vi "白子权值.vi"(0 "当前棋盘状态":i32[][](array[numeric]), 7 "行":dbl, 9 "列":u8) -> (4 "白子总权值":i32)   [LabVIEW 2018]
panel:
  out "活1?右上":bool
  out "活1?左下":bool
  out "活1?左上":bool
  out "活1?右下":bool
  out "活1?正上":bool
  out "活1?正下":bool
  out "活1?正左":bool
  out "活1?正右":bool
  out "3个白子？右上":bool
  out "2个白子？右上":bool
  out "1个白子？右上":bool
  out "3个白子？左下":bool
  out "2个白子？左下":bool
  out "1个白子？ 左下":bool
  out "3个白子？左上":bool
  out "2个白子？左上":bool
  out "1个白子？左上":bool
  out "3个白子？右下":bool
  out "2个白子？右下":bool
  out "1个白子？右下":bool
  out "3个白子？ 正上":bool
  out "2个白子？ 正上":bool
  out "1个白子？ 正上":bool
  out "3个白子？ 正下":bool
  out "2个白子？正下":bool
  out "1个白子？ 正下":bool
  out "3个白子？正左":bool
  out "2个白子？正左":bool
  out "1个白子？正左":bool
  out "3个白子？正右":bool
  out "2个白子？正右":bool
  out "1个白子？正右":bool
  out "右上方向权值":i32
  out "左下方向权值":i32
  out "左上方向权值":i32
  out "右下方向权值":i32
  out "正上方权值":i32
  out "正下方权值":i32
  out "正左方向权值":i32
  out "正右方向权值":i32
  # "0"
  # "1"
  # "2"
  # "3"
  # "4"
  # "5"
  # "6"
  # "7"
  # "8"
  # "9"
  # "10"
  # "11"
  # "12"
  # "13"
  # "14"
  # "0"
  # "1"
  # "2"
  # "3"
  # "4"
  # "5"
  # "6"
  # "7"
  # "8"
  # "9"
  # "10"
  # "11"
  # "12"
  # "13"
  # "14"
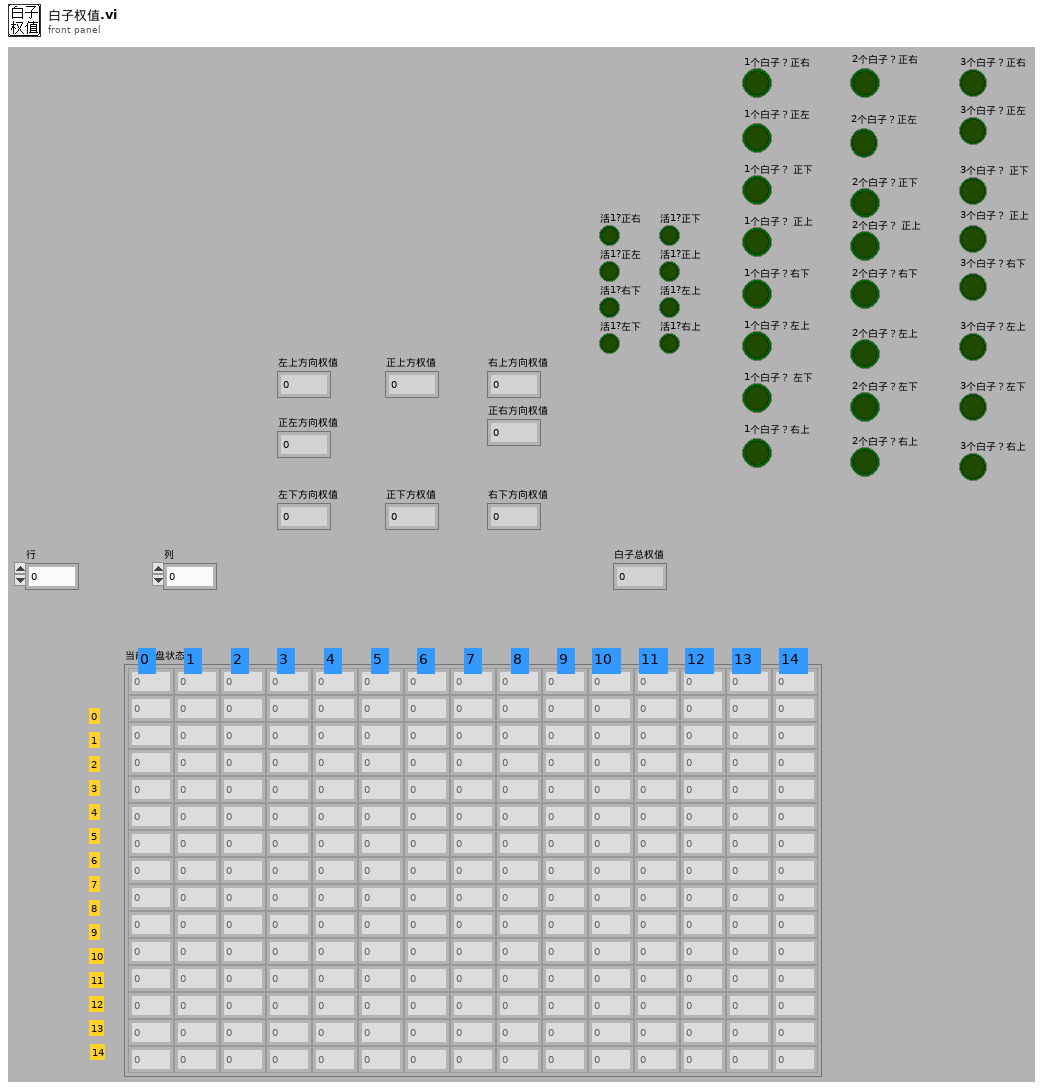
[diagram p1: front panel]
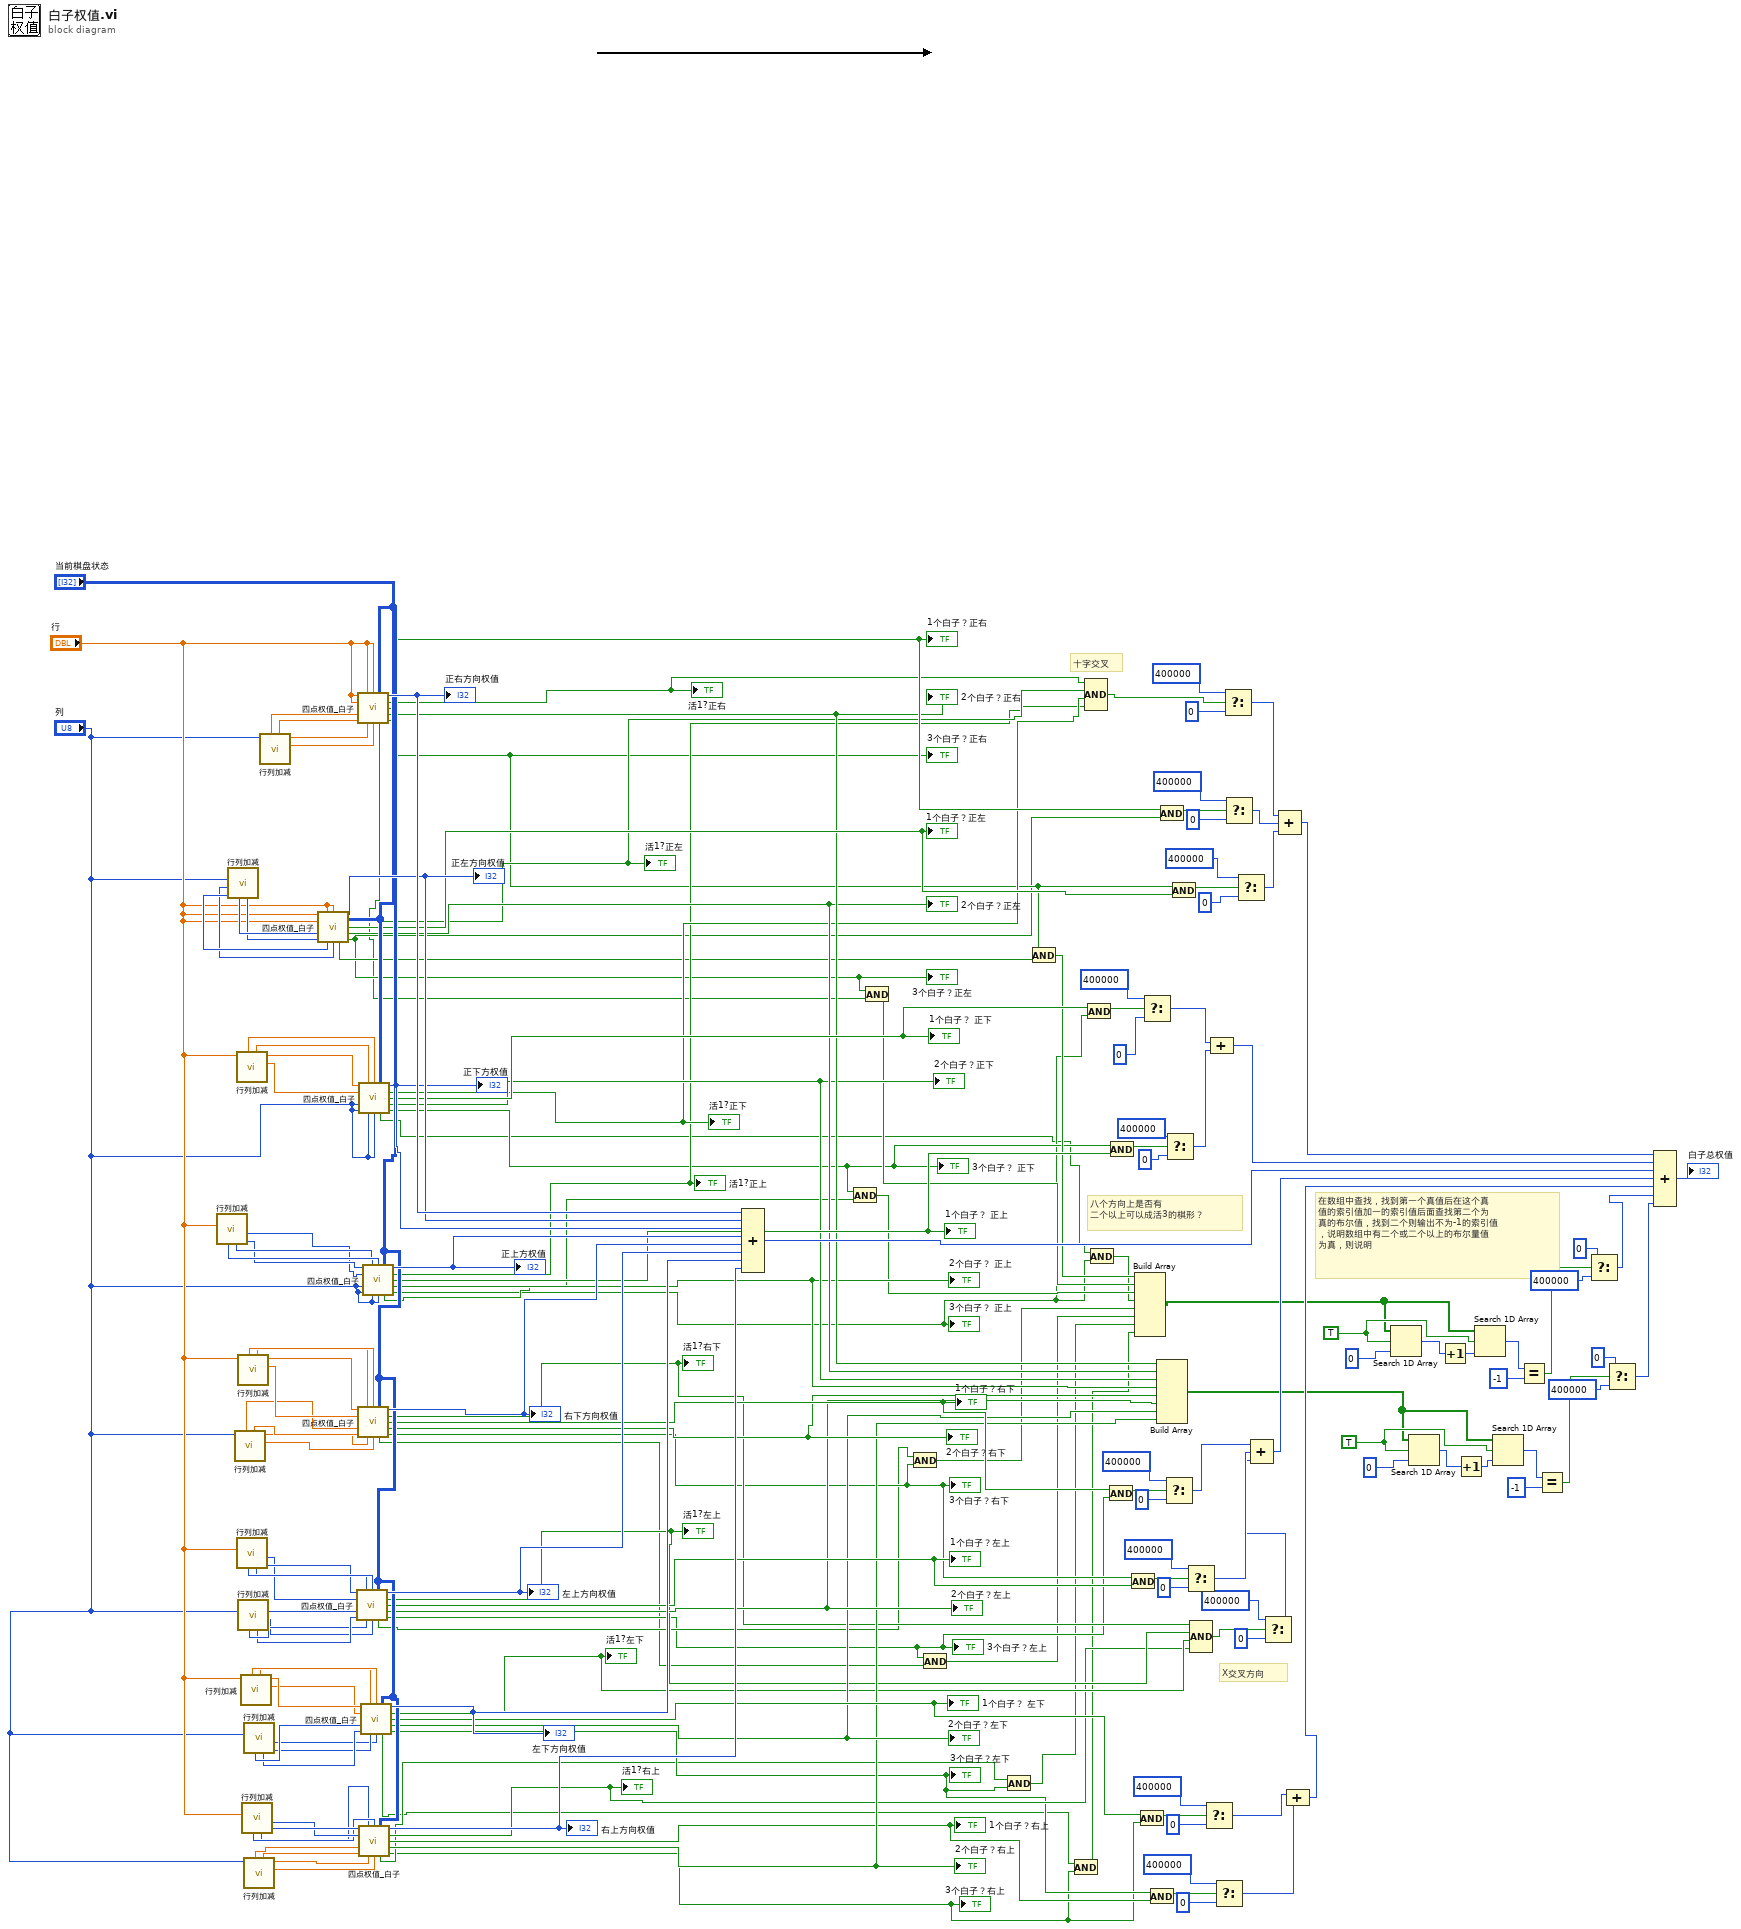
[diagram p0: block diagram]
diagram:
  w49 = TRUE ("element")
  w72 = TRUE ("element")
  # "在数组中查找，找到第一个真值后在这个真\n值的索引值加一的索引值后面查找第二个为\n真的布尔值，找到二个则输出不为-1的索引值\n，说明数组中有二个或二个以上的布尔量值\n为真，则说明"
  # "八个方向上是否有\n二个以上可以成活3的棋形？"
  # "X交叉方向"
  # "十字交叉"
  n1 = call "行列加减.vi"("减"="行") -> ("x-3"=w157:i32, "x-4"=w156:i32, "x-2"=w158:i32, "x-1"=w159:i32)  [unwired: 3 in, 4 out]
  n2 = call "行列加减.vi"("减"="列") -> ("x-3"=w165:i32, "x-4"=w164:i32, "x-2"=w166:i32, "x-1"=w167:i32)  [unwired: 3 in, 4 out]
  n3 = call "行列加减.vi"("加"="列") -> ("x+4"=w148:dbl, "x+3"=w149:dbl, "x+2"=w150:dbl, "x+1"=w151:dbl)  [unwired: 3 in, 4 out]
  n4 = call "行列加减.vi"("加"="行") -> ("x+4"=w160:dbl, "x+3"=w161:dbl, "x+2"=w162:dbl, "x+1"=w163:dbl)  [unwired: 3 in, 4 out]
  n5 = call "行列加减.vi"("减"="行") -> ("x-3"=w144:i32, "x-4"=w143:i32, "x-2"=w145:i32, "x-1"=w146:i32)  [unwired: 3 in, 4 out]
  n6 = call "行列加减.vi"("加"="行") -> ("x+4"=w152:dbl, "x+3"=w153:dbl, "x+2"=w154:dbl, "x+1"=w155:dbl)  [unwired: 3 in, 4 out]
  n7 = call "行列加减.vi"("减"="列") -> ("x-3"=w140:i32, "x-4"=w139:i32, "x-2"=w141:i32, "x-1"=w142:i32)  [unwired: 3 in, 4 out]
  n8 = call "行列加减.vi"("加"="行") -> ("x+4"=w134:dbl, "x+3"=w135:dbl, "x+2"=w136:dbl, "x+1"=w137:dbl)  [unwired: 3 in, 4 out]
  n9 = call "行列加减.vi"("减"="行") -> ("x-3"=w125:i32, "x-4"=w124:i32, "x-2"=w117:i32, "x-1"=w118:i32)  [unwired: 3 in, 4 out]
  n10 = call "行列加减.vi"("减"="列") -> ("x-3"=w131:i32, "x-4"=w130:i32, "x-2"=w132:i32, "x-1"=w133:i32)  [unwired: 3 in, 4 out]
  n11 = call "行列加减.vi"("加"="列") -> ("x+4"=w120:dbl, "x+3"=w121:dbl, "x+2"=w122:dbl, "x+1"=w123:dbl)  [unwired: 3 in, 4 out]
  n12 = call "行列加减.vi"("加"="列") -> ("x+4"=w168:dbl, "x+3"=w169:dbl, "x+2"=w170:dbl, "x+1"=w171:dbl)  [unwired: 3 in, 4 out]
  n13 = call "四点权值_白子.vi"("3位置行"="行", "2位置行"="行", "1位置行"="行", "当前棋盘状态"="当前棋盘状态", "4位置行"="行", "1位置列"=w167, "2位置列"=w166, "3位置列"=w165, "4位置列"=w164) -> ("白子四位置权值"=w174:i32, "有2个白子?或白子加无子?"=w41:bool, "第1个是白子？"=w108:bool, "3个白子?"=w61:bool, "第一个位置为空？"=w23:bool, "3个白子？或2个白子加无子"=w21:bool)  [unwired: 1 in]
  "正左方向权值" <- w174
  "1个白子？正左" <- w108
  "2个白子？正左" <- w61
  "3个白子？正左" <- w21
  "活1?正左" <- w41
  n14 = call "四点权值_白子.vi"("3位置行"=w144, "2位置行"=w145, "1位置行"=w146, "当前棋盘状态"="当前棋盘状态", "4位置行"=w143, "1位置列"=w142, "2位置列"=w141, "3位置列"=w140, "4位置列"=w139) -> ("白子四位置权值"=w138:i32, "有2个白子?或白子加无子?"=w33:bool, "第1个是白子？"=w86:bool, "3个白子?"=w57:bool, "第一个位置为空？"=w14:bool, "3个白子？或2个白子加无子"=w12:bool)  [unwired: 1 in]
  "左上方向权值" <- w138
  "1个白子？左上" <- w86
  "2个白子？左上" <- w57
  "3个白子？左上" <- w12
  "活1?左上" <- w33
  n15 = call "四点权值_白子.vi"("3位置行"="行", "2位置行"="行", "1位置行"="行", "当前棋盘状态"="当前棋盘状态", "4位置行"="行", "1位置列"=w171, "2位置列"=w170, "3位置列"=w169, "4位置列"=w168) -> ("白子四位置权值"=w175:i32, "有2个白子?或白子加无子?"=w26:bool, "第1个是白子？"=w112:bool, "3个白子?"=w62:bool, "第一个位置为空？"=w20:bool, "3个白子？或2个白子加无子"=w24:bool)  [unwired: 1 in]
  "正右方向权值" <- w175
  "1个白子？正右" <- w112
  "2个白子？正右" <- w62
  "3个白子？正右" <- w24
  "活1?正右" <- w26
  n16 = call "四点权值_白子.vi"("3位置行"=w153, "2位置行"=w154, "1位置行"=w155, "当前棋盘状态"="当前棋盘状态", "4位置行"=w152, "1位置列"=w151, "2位置列"=w150, "3位置列"=w149, "4位置列"=w148) -> ("白子四位置权值"=w147:i32, "有2个白子?或白子加无子?"=w34:bool, "第1个是白子？"=w91:bool, "3个白子?"=w58:bool, "第一个位置为空？"=w11:bool, "3个白子？或2个白子加无子"=w15:bool)  [unwired: 1 in]
  "右下方向权值" <- w147
  "1个白子？右下" <- w91
  "2个白子？右下" <- w58
  "3个白子？右下" <- w15
  "活1?右下" <- w34
  n17 = call "四点权值_白子.vi"("3位置行"=w161, "2位置行"=w162, "1位置行"=w163, "当前棋盘状态"="当前棋盘状态", "4位置行"=w160, "1位置列"="列", "2位置列"="列", "3位置列"="列", "4位置列"="列") -> ("白子四位置权值"=w173:i32, "有2个白子?或白子加无子?"=w40:bool, "第1个是白子？"=w102:bool, "3个白子?"=w60:bool, "第一个位置为空？"=w1:bool, "3个白子？或2个白子加无子"=w18:bool)  [unwired: 1 in]
  "正下方权值" <- w173
  "1个白子？ 正下" <- w102
  "2个白子？正下" <- w60
  "3个白子？ 正下" <- w18
  "活1?正下" <- w40
  n18 = call "四点权值_白子.vi"("3位置行"=w125, "2位置行"=w117, "1位置行"=w118, "当前棋盘状态"="当前棋盘状态", "4位置行"=w124, "1位置列"=w123, "2位置列"=w122, "3位置列"=w121, "4位置列"=w120) -> ("白子四位置权值"=w119:i32, "有2个白子?或白子加无子?"=w31:bool, "第1个是白子？"=w25:bool, "3个白子?"=w55:bool, "第一个位置为空？"=w7:bool, "3个白子？或2个白子加无子"=w6:bool)  [unwired: 1 in]
  "右上方向权值" <- w119
  "1个白子？右上" <- w25
  "2个白子？右上" <- w55
  "3个白子？右上" <- w6
  "活1?右上" <- w31
  n19 = call "四点权值_白子.vi"("3位置行"=w135, "2位置行"=w136, "1位置行"=w137, "当前棋盘状态"="当前棋盘状态", "4位置行"=w134, "1位置列"=w133, "2位置列"=w132, "3位置列"=w131, "4位置列"=w130) -> ("白子四位置权值"=w129:i32, "有2个白子?或白子加无子?"=w32:bool, "第1个是白子？"=w79:bool, "3个白子?"=w56:bool, "第一个位置为空？"=w5:bool, "3个白子？或2个白子加无子"=w8:bool)  [unwired: 1 in]
  "左下方向权值" <- w129
  "1个白子？ 左下" <- w79
  "2个白子？左下" <- w56
  "3个白子？左下" <- w8
  "活1?左下" <- w32
  n20 = call "四点权值_白子.vi"("3位置行"=w157, "2位置行"=w158, "1位置行"=w159, "当前棋盘状态"="当前棋盘状态", "4位置行"=w156, "1位置列"="列", "2位置列"="列", "3位置列"="列", "4位置列"="列") -> ("白子四位置权值"=w172:i32, "有2个白子?或白子加无子?"=w39:bool, "第1个是白子？"=w98:bool, "3个白子?"=w59:bool, "第一个位置为空？"=w17:bool, "3个白子？或2个白子加无子"=w2:bool)  [unwired: 1 in]
  "正上方权值" <- w172
  "1个白子？ 正上" <- w98
  "2个白子？ 正上" <- w59
  "3个白子？ 正上" <- w2
  "活1?正上" <- w39
  n21 = Compound Arithmetic op=ADD(w175, w174, w173, w172, w147, w138, w129, w119) -> (w95:i32)
  n22 = And(x=w18, y=w17) -> (x .and. y?=w16:bool)
  n23 = And(x=w21, y=w20) -> (x .and. y?=w19:bool)
  n24 = And(x=w14, y=w15) -> (x .and. y?=w13:bool)
  n25 = And(x=w12, y=w11) -> (x .and. y?=w10:bool)
  n26 = And(x=w7, y=w8) -> (x .and. y?=w9:bool)
  n27 = And(x=w24, y=w23) -> (x .and. y?=w22:bool)
  n28 = And(x=w5, y=w6) -> (x .and. y?=w4:bool)
  n29 = And(x=w102, y=w2) -> (x .and. y?=w105:bool)
  n30 = Compound Arithmetic op=AND(w26, w41, w40, w39) -> (w36:bool)
  n31 = And(x=w1, y=w2) -> (x .and. y?=w3:bool)
  n32 = And(x=w91, y=w12) -> (x .and. y?=w92:bool)
  n33 = And(x=w18, y=w98) -> (x .and. y?=w101:bool)
  n34 = And(x=w15, y=w86) -> (x .and. y?=w89:bool)
  n35 = Build Array(w22, w19, w16, w3, w13, w10, w9, w4) -> (w69:bool[])
  n36 = And(x=w79, y=w6) -> (x .and. y?=w83:bool)
  n37 = Select(t=400000, s=w105, f=0) -> (s? t:f=w63:i32)
  n38 = And(x=w8, y=w25) -> (x .and. y?=w75:bool)
  n39 = And(x=w112, y=w21) -> (x .and. y?=w114:bool)
  n40 = Build Array(w62, w61, w60, w59, w58, w57, w56, w55) -> (w47:bool[])
  n41 = Select(t=400000, s=w92, f=0) -> (s? t:f=w90:i32)
  n42 = Select(t=400000, s=w101, f=0) -> (s? t:f=w97:i32)
  n43 = And(x=w24, y=w108) -> (x .and. y?=w111:bool)
  n44 = Select(t=400000, s=w89, f=0) -> (s? t:f=w85:i32)
  n45 = Compound Arithmetic op=AND(w34, w33, w32, w31) -> (w29:bool)
  n46 = Select(t=400000, s=w83, f=0) -> (s? t:f=w78:i32)
  n47 = Compound Arithmetic op=ADD(w63, w97) -> (w96:i32)
  n48 = Select(t=400000, s=w75, f=0) -> (s? t:f=w74:i32)
  n49 = Select(t=400000, s=w36, f=0) -> (s? t:f=w35:i32)
  n50 = Select(t=400000, s=w114, f=0) -> (s? t:f=w113:i32)
  n51 = Select(t=400000, s=w111, f=0) -> (s? t:f=w107:i32)
  n52 = Select(t=400000, s=w29, f=0) -> (s? t:f=w27:i32)
  n53 = Compound Arithmetic op=ADD(w90, w85, w27) -> (w84:i32)
  n54 = Compound Arithmetic op=ADD(w35, w113, w107) -> (w106:i32)
  n55 = Compound Arithmetic op=ADD(w78, w74) -> (w80:i32)
  n56 = Search 1D Array(1D array=w69, element=w72, start index (0)=0) -> (index of element=w44:i32)
  n57 = Search 1D Array(1D array=w47, element=w49, start index (0)=0) -> (index of element=w42:i32)
  n58 = Increment(x=w44) -> (x+1=w45:i32)
  n59 = Increment(x=w42) -> (x+1=w43:i32)
  n60 = Search 1D Array(1D array=w69, element=w72, start index (0)=w45) -> (index of element=w71:i32)
  n61 = Search 1D Array(1D array=w47, element=w49, start index (0)=w43) -> (index of element=w50:i32)
  n62 = Equal?(x=w71, y=-1) -> (x = y?=w67:bool)
  n63 = Equal?(x=w50, y=-1) -> (x = y?=w53:bool)
  n64 = Select(t=0, s=w67, f=400000) -> (s? t:f=w66:i32)
  n65 = Select(t=0, s=w53, f=400000) -> (s? t:f=w46:i32)
  n66 = Compound Arithmetic op=ADD(w106, w96, w95, w84, w80, w66, w46) -> (→"白子总权值":i32)
